vi "Curtin1_Search.vi"(9 "Old Files":T3[](array[typedef])) -> (1 "New Files":T3[](array[typedef]), 3 "Ok?":bool)   [LabVIEW 2022 SP3]
uses:
  Curtin1_Label.ctl
  <vilib>/Utility/miscctls.llb/LVSelectionTypeDef.ctl
panel:
  in  "Listing Order":T1(ring)
  in  "Tags":T2={"Pattern (eg. H,V)"="H,V", "File type"={"AvR"=TRUE, "AvC"=FALSE, "trf"=FALSE, "wav"=FALSE, "All"=FALSE}, "keywords 1"="", "keywords 2"="", "keywords 3"=""}
  out "# Files":i32
  out "AllFiles":path[](array[path])
  in  "Options":i32[](listbox)
  out "Files":path[](array[path])
  in  "Dialog":bool
  out "Subfolder":string
  in  "Search":bool
  out "Folder":cluster{"Folder Path":path, "tags":string[]}[](array[cluster])
  out "List":string
  in  "Cancel Button":bool
  in  "OK Button":bool
  # "Or"
  # "Or"
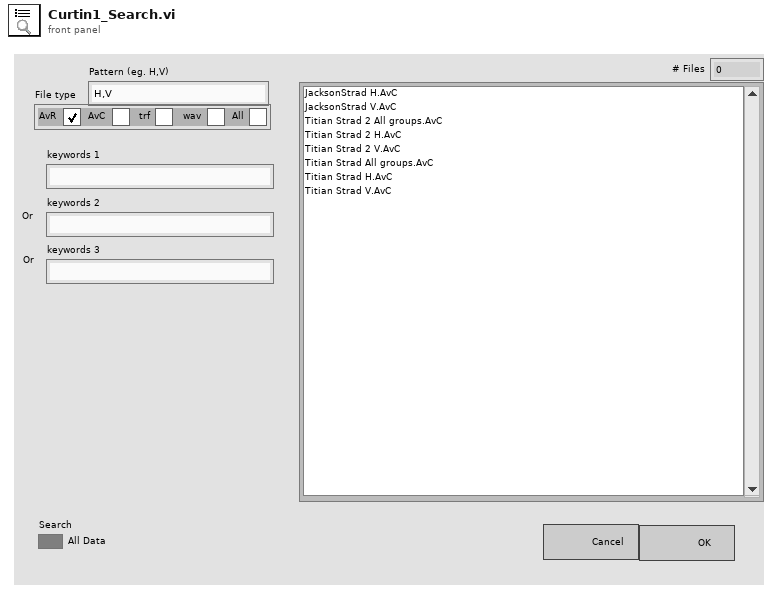
[diagram p1: front panel]
types:
  T1 = enum16{"Alphabetical", "Chronological", "Hit Strength (min to max)", "Hit Strength (max to min)"}
  T2 = cluster{"Pattern (eg. H,V)":string, "File type":cluster{"AvR":bool, "AvC":bool, "trf":bool, "wav":bool, "All":bool}, "keywords 1":string, "keywords 2":string, "keywords 3":string}
  T3 = typedef "Curtin1_Label.ctl" = cluster{"Show?":bool, "Name":string, "Color":u32, "Path":path, "Show Notes":bool}
  T4 = typedef "LVSelectionTypeDef.ctl" = cluster{"Selection Start":u32, "Selection End":u32}
  T5 = cluster{"Pattern (eg. H,V)":string, "File type":cluster{"AvR":bool, "AvC":bool, "trf":bool, "wfm":bool, "All":bool}, "keywords 1":string, "keywords 2":string, "keywords 3":string}
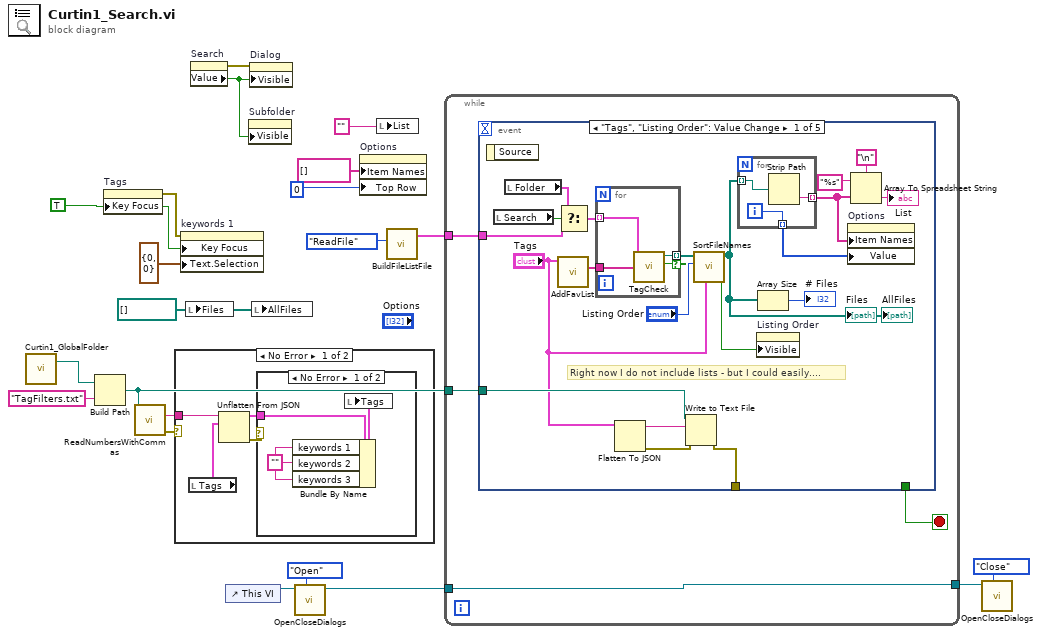
[diagram p0: block diagram]
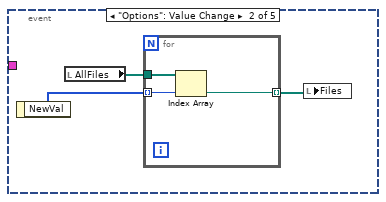
[diagram p4: hidden frame]
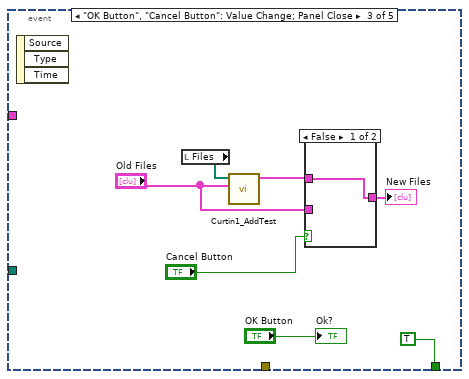
[diagram p5: hidden frame]
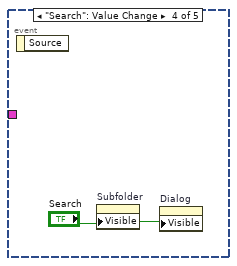
[diagram p7: hidden frame]
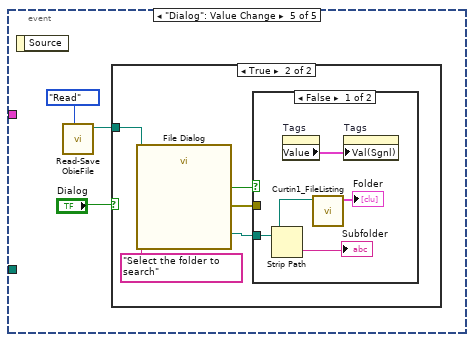
[diagram p8: hidden frame]
diagram:
  w1 = path[] [] ("Files")
  w11 = TRUE ("Visible")
  n1 = call "Curtin1_GlobalFolder.vi"() -> ("LabVIEW Data Path"=w19:path)  [unwired: 1 in, 1 out]
  n2 = Build Path(base path=w19, name or relative path="TagFilters.txt") -> (appended path=w9:path)
  n3 = property on="Tags" class="Clust (strict)"("Key Focus"=w11) -> (error out=w10:errorcluster)  [unwired: 2 in, 1 out]
  n4 = call "ReadNumbersWithCommas.vi"("file (use dialog)"=w9) -> ("error out"=w7:errorcluster, "text"=w8:string)  [unwired: 7 in, 2 out]
  n5 = case shown="No Error" w7 {
    tunnel: w8 -> [w24 _]
    frame No Error {
      n6 = local read "Tags"() -> (w25:T2)
      n7 = Unflatten From JSON(JSON string=w24, type and defaults=w25) -> (value=w22:T2, error out=w23:errorcluster)  [unwired: 5 in]
      n8 = case shown="No Error" w23 {
        tunnel: w22 -> [w28 _]
        frame No Error {
          w27 = "" ("Tags 1")
          n9 = Bundle By Name(cluster=w28, "keywords 1"=w27, "keywords 2"=w27, "keywords 3"=w27) -> (w26:T2)
          n10 = local write "Tags"(w26) -> ()
        }
        frame Error {
        }
      }
    }
    frame Error {
    }
  }
  n11 = property on="keywords 1" class="Str"(error in=w10, "Key Focus"=w11, "Text.Selection"=T4 {"Selection Start"=0, "Selection End"=0}) -> ()  [unwired: 1 in, 2 out]
  n12 = local write "Files"(w1) -> ()
  n13 = property on="Search" class="Bool (strict)"() -> (error out=w15:errorcluster, "Value"=w14:bool)  [unwired: 2 in, 1 out]
  n14 = control-ref of="This VI"() -> (w5:refnum<vi>)
  n15 = property on="Subfolder" class="Str"("Visible"=w14) -> ()  [unwired: 2 in, 2 out]
  n16 = property on="Dialog" class="Bool"(error in=w15, "Visible"=w14) -> ()  [unwired: 1 in, 2 out]
  n17 = local write "AllFiles"(w1) -> ()
  n18 = call "OpenCloseDialogs.vi"("Task"=enum16{"Open", "Close"}."Open", "VI in"=w5) -> ("VI out"=w2:refnum<vi>)  [unwired: 8 in, 1 out]
  n19 = property on="Options" class="LstBox (strict)"("Item Names"=string[] [], "Top Row"=0) -> ()  [unwired: 2 in, 2 out]
  n20 = local write "List"("" ("List")) -> ()
  n21 = call "BuildFileListFile.vi"("Task"=enum16{"BuildFile", "ReadFile"}."ReadFile") -> ("Instruments"=w16:cluster{"Folder Path":path, "tags":string[]}[])  [unwired: 9 in, 1 out]
  n22 = while {
    tunnel: w16 -> [w31]
    tunnel: w9 -> [w30]
    tunnel: [w29] -> w3
    tunnel: w2 -> [w29]
    stop <- w32 stop-if-true
    n23 = event shown="[0] \"Tags\", \"Listing Order\": Value Change" {
      selector: _ -> [_ _ _ _ _]
      dyn-events: _ -> [_ _ _ _ _]
      timeout: _ -> [_ _ _ _ _]
      tunnel: [_ _ TRUE _ _] -> w32
      tunnel: w31 -> [w40 _ _ _ _]
      tunnel: w30 -> [w46 _ _ _ _]
      tunnel: [w44 _ _ _ _] -> _
      event "Tags", "Listing Order": Value Change {
        # "Right now I do not include lists - but I could easily...."
        n24 = event-data() -> ()  [unwired: 1 in, 1 out]
        n25 = local read "Search"() -> (w41:bool)
        n26 = local read "Folder"() -> (w39:cluster{"Folder Path":path, "tags":string[]}[])
        n27 = call "AddFavList.vi"("Tags"="Tags") -> ("Tags"=w51:string[])  [unwired: 8 in, 2 out]
        n28 = Select(t=w39, s=w41, f=w40) -> (s? t:f=w38:cluster{"Folder Path":path, "tags":string[]}[])
        n29 = for {
          tunnel: w51 -> [w57]
          tunnel: [w59] -> w37 mode=indexing if=w58
          tunnel: w38 -> [w56] mode=indexing
          n30 = call "TagCheck.vi"("Tags"=w57, 11:w56) -> ("Good?"=w58:bool, "Path out"=w59:path)  [unwired: 8 in]
        }
        n31 = Flatten To JSON(anything="Tags") -> (JSON string=w47:string, 11:w45:errorcluster)  [unwired: 2 in]
        n32 = Write to Text File(file (use dialog)=w46, text=w47, error in=w45) -> (error out=w44:errorcluster)  [unwired: 1 in, 2 out]
        n33 = call "SortFileNames.vi"("Tags"="Tags", "Listing Order"="Listing Order", "Files in"=w37) -> ("wfm only?"=w33:bool, "Files out"=w36:path[])  [unwired: 7 in]
        "Files" <- w36
        "AllFiles" <- w36
        n34 = for {
          tunnel: w36 -> [w55] mode=indexing
          tunnel: [w54] -> w43 mode=indexing
          tunnel: [w53] -> w42 mode=indexing
          i -> [w53]
          n35 = Strip Path(path=w55) -> (name=w54:string)  [unwired: 1 out]
        }
        n36 = property on="Listing Order" class="Enum (strict)"("Visible"=w33) -> ()  [unwired: 2 in, 2 out]
        n37 = Array Size(array=w36) -> (size(s)=→"# Files":i32)
        n38 = property on="Options" class="LstBox (strict)"("Item Names"=w43, "Value"=w42) -> ()  [unwired: 2 in, 2 out]
        n39 = Array To Spreadsheet String(delimiter (Tab)="\n", array=w43, 3:"%s" ("format string")) -> (spreadsheet string=→"List":string)
      }
      event "Options": Value Change {
        n40 = event-data() -> ("NewVal"=w61:i32[])  [unwired: 1 in]
        n41 = local read "AllFiles"() -> (w62:path[])
        n42 = for {
          tunnel: w62 -> [w65]
          tunnel: w61 -> [w64] mode=indexing
          tunnel: [w63] -> w60 mode=indexing
          n43 = Index Array(array=w65, index=w64) -> (element=w63:path)
        }
        n44 = local write "Files"(w60) -> ()
      }
      event "OK Button", "Cancel Button": Value Change; Panel Close {
        n45 = event-data() -> ()  [unwired: 1 in, 3 out]
        n46 = local read "Files"() -> (w72:path[])
        n47 = call "Curtin1_AddTest.vi"("Old Files"="Old Files", "Selected Paths"=w72) -> ("New Files"=w69:T3[])  [unwired: 9 in]
        n48 = case shown="False" "Cancel Button" {
          tunnel: "Old Files" -> [_ w74]
          tunnel: w69 -> [w73 _]
          tunnel: [w73 w74] -> w68
          frame False {
          }
          frame True {
          }
        }
        "New Files" <- w68
        "Ok?" <- "OK Button"
      }
      event "Search": Value Change {
        n49 = event-data() -> ()  [unwired: 1 in, 1 out]
        n50 = property on="Subfolder" class="Str"("Visible"="Search") -> ()  [unwired: 2 in, 2 out]
        n51 = property on="Dialog" class="Bool"("Visible"="Search") -> ()  [unwired: 2 in, 2 out]
      }
      event "Dialog": Value Change {
        n52 = event-data() -> ()  [unwired: 1 in, 1 out]
        n53 = call "Read-Save ObieFile.vi"("Task"=enum16{"Save", "Read"}."Read") -> ("DataPath Out"=w76:path)  [unwired: 8 in, 2 out]
        n54 = case shown="True" "Dialog" {
          tunnel: w76 -> [_ w80]
          frame False {
          }
          frame True {
            n55 = call "File Dialog"("start path"=w80, "prompt"="Select the folder to search" ("List")) -> ("selected path"=w83:path, "cancelled"=w82:bool, "error out"=w81:errorcluster)  [unwired: 10 in, 1 out]
            n56 = case shown="False" w82 {
              tunnel: w83 -> [w86 _]
              tunnel: w81 -> [_ _]
              frame False {
                n57 = Strip Path(path=w86) -> (name=→"Subfolder":string)  [unwired: 1 out]
                n58 = property on="Tags" class="Clust (strict)"() -> ("Value"=w84:T5)  [unwired: 2 in, 2 out]
                n59 = call "Curtin1_FileListing.vi"("Folder Path"=w86) -> ("Array"=→"Folder":cluster{"Folder Path":path, "tags":string[]}[])  [unwired: 10 in]
                n60 = property on="Tags" class="Clust (strict)"("Val(Sgnl)"=w84) -> ()  [unwired: 2 in, 2 out]
              }
              frame True {
              }
            }
          }
        }
      }
    }
  }
  n61 = call "OpenCloseDialogs.vi"("Task"=enum16{"Open", "Close"}."Close", "VI in"=w3) -> ()  [unwired: 8 in, 2 out]
